vi "Configure Clock Gate Delay.vi"(6 "Time Mode Gate Delay (2.67E-8 s)":dbl=2.67e-08, 7 "Clock Mode Gate Delay (1)":u32=1, 8 "error in (no error)":errorcluster, 9 "Gate Delay Operating Mode (0: Time)":i32(ring) items=["Time", "Clock"], 10 "Enable Clock Gate Delay (F: Disable)":bool, 11 "VISA resource name":refnum<visa-resource-name>) -> (0 "error out":errorcluster, 3 "VISA resource name out":refnum<visa-resource-name>)   [LabVIEW 2018, in "Agilent PSG MXG Series.lvlib"]
doc: "Configures the gate signal's delay function.\n\n<b>Notes:</b>\n(1) It is applicable for N5172B/82B with <b>Option UN7</b> only.\n(2) It is valid only when the gate is enabled that in <b>Enable Clock Gate.vi</b>."
uses:
  Agilent PSG MXG Series.lvlib
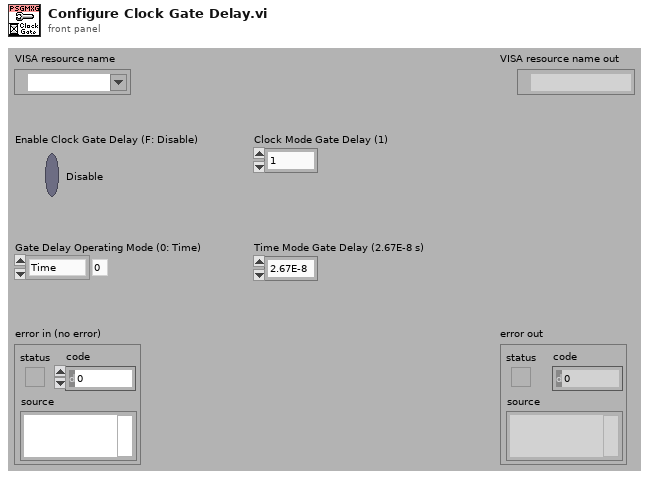
[diagram p1: front panel]
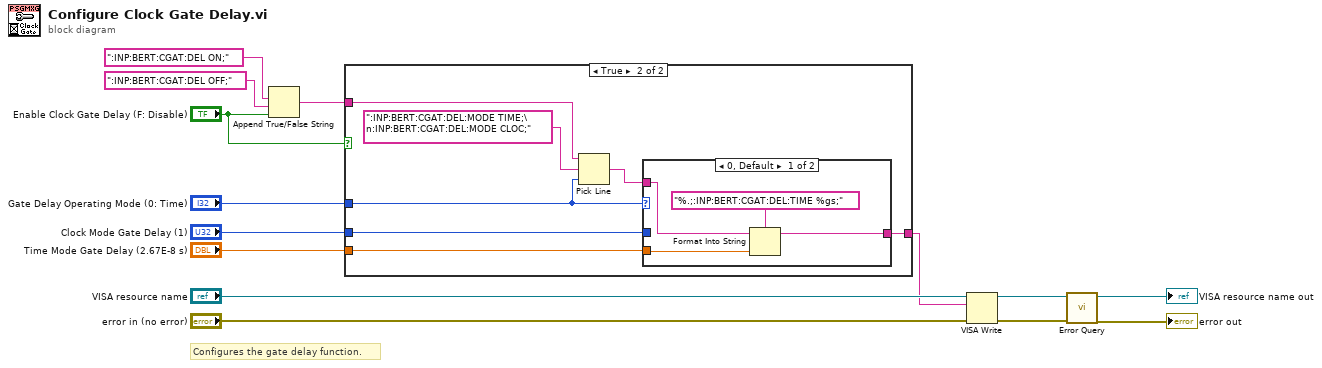
[diagram p0: block diagram]
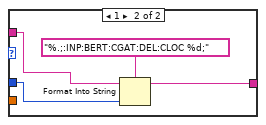
[diagram p3: hidden frame]
diagram:
  # "Configures the gate delay function."
  n1 = Append True/False String(1:"Enable Clock Gate Delay (F: Disable)", 2:":INP:BERT:CGAT:DEL OFF;", 3:":INP:BERT:CGAT:DEL ON;") -> (0:w6:string)  [unwired: 1 in]
  n2 = case shown="True" "Enable Clock Gate Delay (F: Disable)" {
    tunnel: "Time Mode Gate Delay (2.67E-8 s)" -> [_ w19]
    tunnel: "Clock Mode Gate Delay (1)" -> [_ w17]
    tunnel: w6 -> [w15 w22]
    tunnel: [w15 w18] -> w2
    tunnel: "Gate Delay Operating Mode (0: Time)" -> [_ w16]
    frame False {
    }
    frame True {
      n3 = Pick Line(string ("")=w22, multi-line string=":INP:BERT:CGAT:DEL:MODE TIME;\n:INP:BERT:CGAT:DEL:MODE CLOC;", line index=w16) -> (output string=w20:string)
      n4 = case shown="0, Default" w16 {
        tunnel: w20 -> [w25 w29]
        tunnel: w19 -> [w24 _]
        tunnel: [w23 w27] -> w18
        tunnel: w17 -> [_ w28]
        frame 0, Default {
          n5 = Format Into String(format string="%.;:INP:BERT:CGAT:DEL:TIME %gs;", initial string=w25, w24) -> (resulting string=w23:string)  [unwired: 1 in, 1 out]
        }
        frame 1 {
          n6 = Format Into String(format string="%.;:INP:BERT:CGAT:DEL:CLOC %d;", initial string=w29, w28) -> (resulting string=w27:string)  [unwired: 1 in, 1 out]
        }
      }
    }
  }
  n7 = VISA Write(VISA resource name="VISA resource name", write buffer=w2, error in (no error)="error in (no error)") -> (VISA resource name out=w12:refnum<visa-resource-name>, error out=w11:errorcluster)  [unwired: 1 out]
  n8 = call "Error Query.vi"("error in (no error)"=w11, "VISA resource name"=w12) -> ("error out"=→"error out":errorcluster, "VISA resource name out"=→"VISA resource name out":refnum<visa-resource-name>)  [unwired: 6 in, 2 out]
